vi "Blinking feature.vi"() -> ()   [LabVIEW 2024]
panel:
  in  "stop":bool
  in  "Numeric":dbl
  # "Overview:\nIn this VI, when you click the cursor in the number, the blink wont happen but when you leave the nu,meric there is a light blinked."
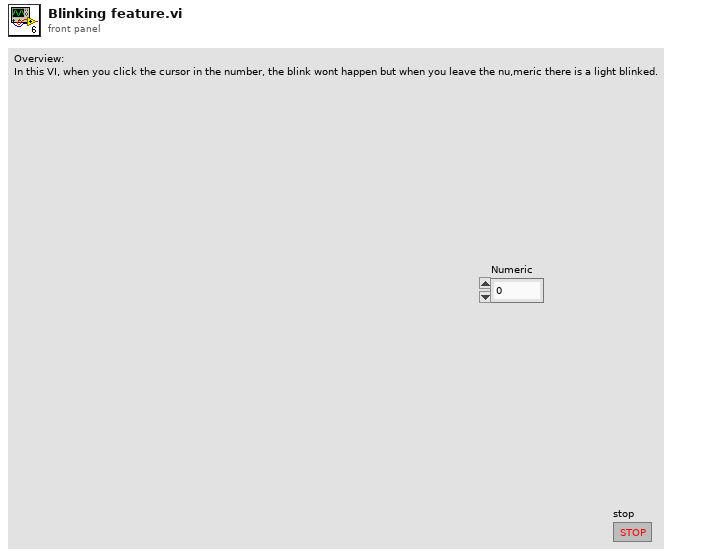
[diagram p1: front panel]
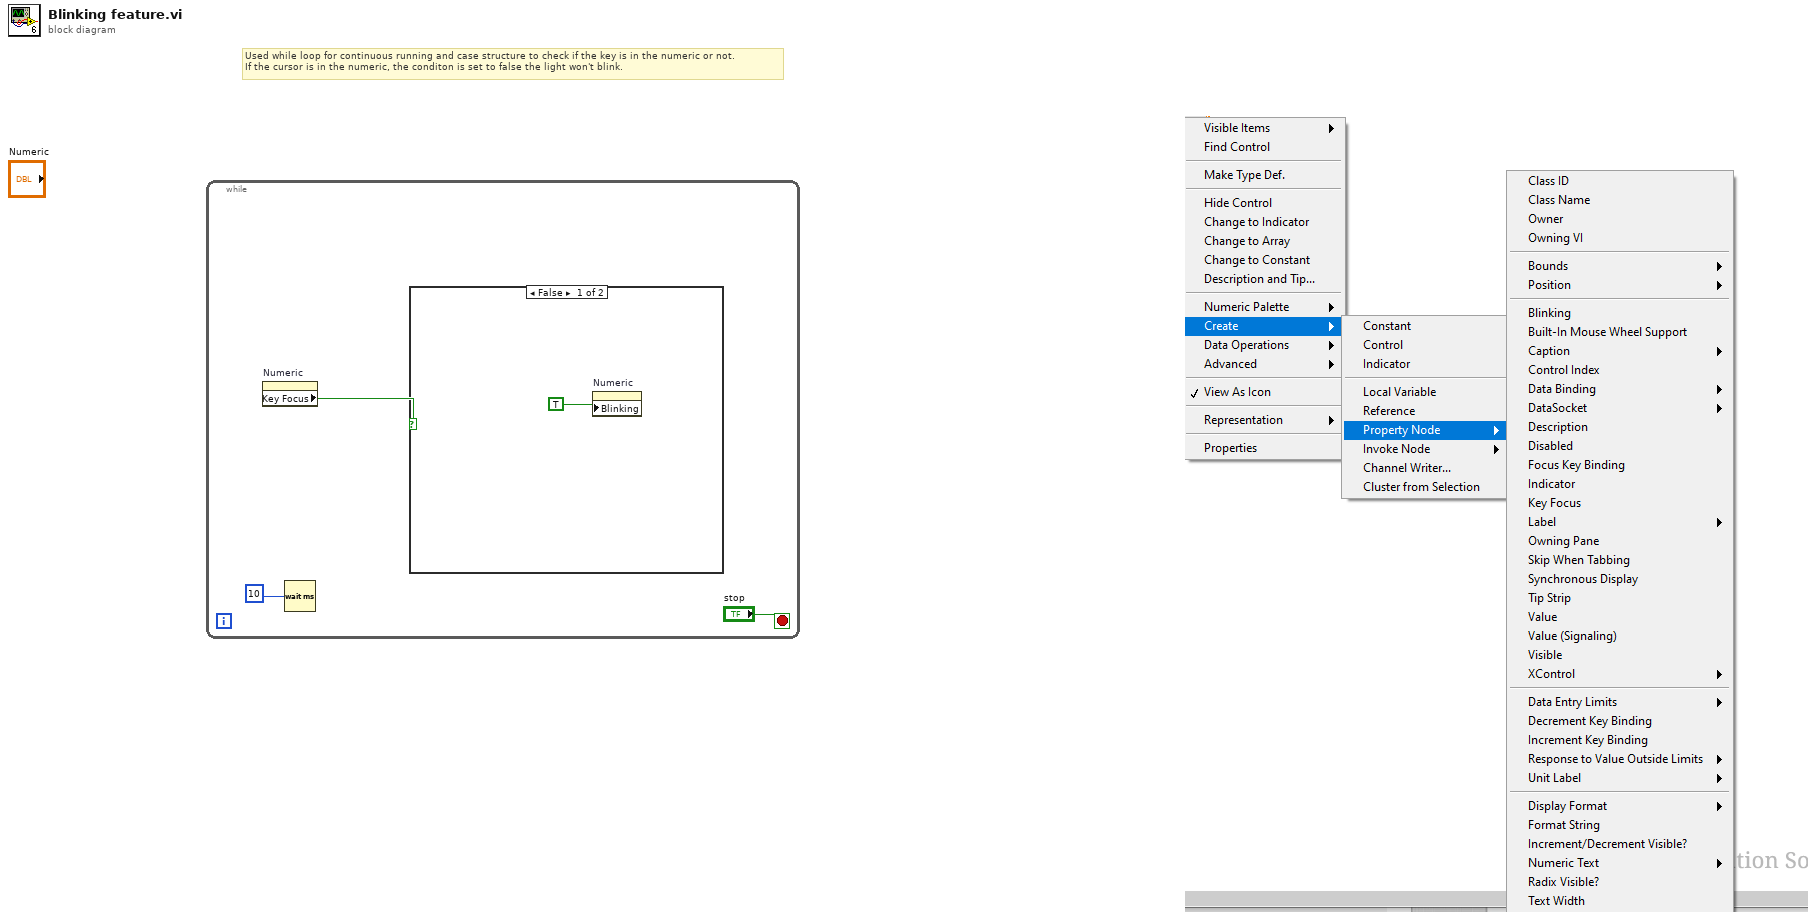
[diagram p0: block diagram]
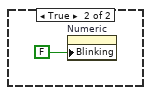
[diagram p2: hidden frame]
diagram:
  # "Used while loop for continuous running and case structure to check if the key is in the numeric or not.\nIf the cursor is in the numeric, the conditon is set to false the light won't blink."
  n1 = while {
    stop <- "stop" stop-if-true
    n2 = property on="Numeric" class="DigNum (strict)"() -> ("Key Focus"=w1:bool)  [unwired: 2 in, 2 out]
    n3 = Wait (ms)(milliseconds to wait=u32 10 ("millisecond timer value")) -> ()  [unwired: 1 out]
    n4 = case shown="False" w1 {
      frame False {
        n5 = property on="Numeric" class="DigNum (strict)"("Blinking"=TRUE) -> ()  [unwired: 2 in, 2 out]
      }
      frame True {
        n6 = property on="Numeric" class="DigNum (strict)"("Blinking"=FALSE) -> ()  [unwired: 2 in, 2 out]
      }
    }
  }
